vi "ShooterManualFlyWheel.vi"(11 "Cluster":T1) -> ()   [LabVIEW 2015]
doc: "call on constants for shooting and give them to the respective motors"
uses:
  constants/constants.ctl
  <vilib>/Rock Robotics/SystemInterfaces/DIO/FPGA_DIOPWMChannel.ctl
  <vilib>/Rock Robotics/WPI/Solenoid/WPI_SolenoidChannel.ctl
panel:
  # "ShooterMotors"
  # "DriveMotors- CAN Bus"
  # "PWM"
  # "ClimberMotors"
  # "CAN Bus"
  # "Pnematic"
  # "PWM"
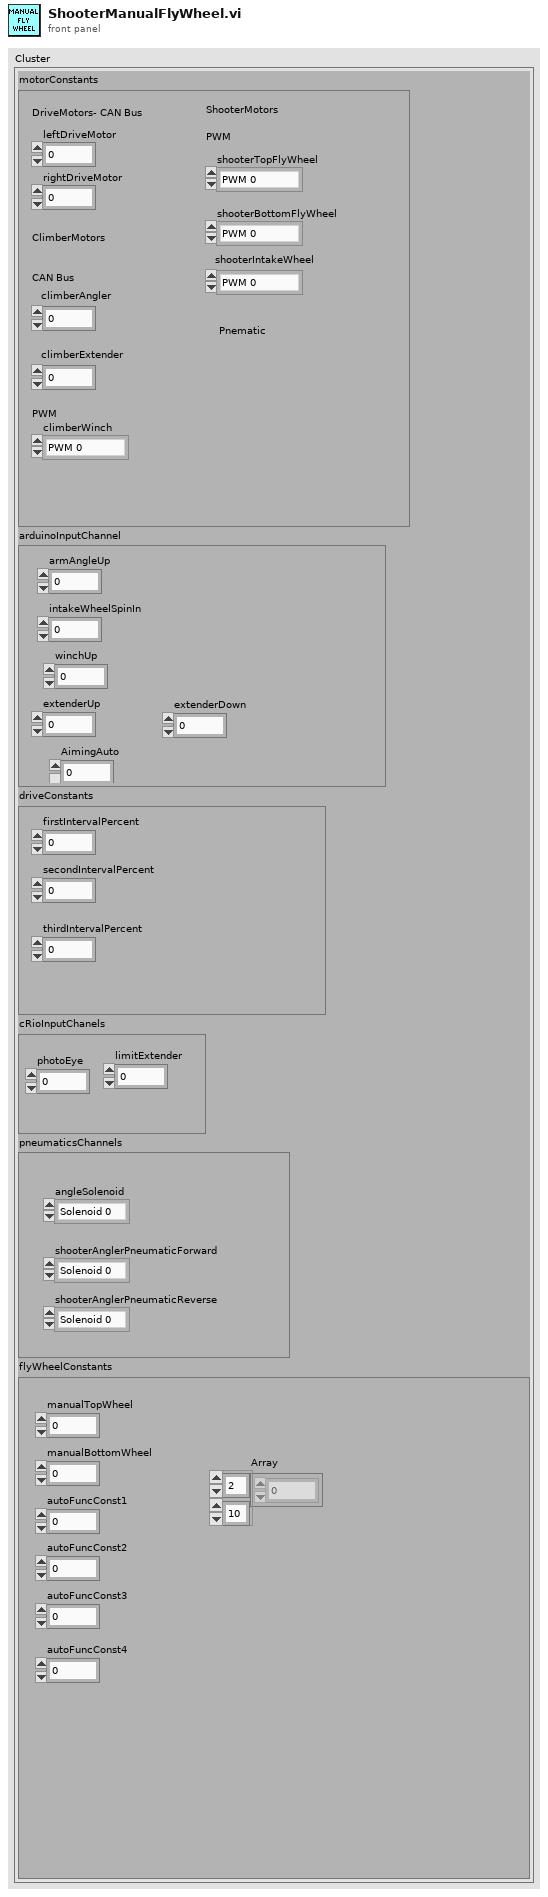
[diagram p1: front panel]
types:
  T1 = typedef "constants.ctl" = cluster{"motorConstants":cluster{"leftDriveMotor":i32, "rightDriveMotor":i32, "climberAngler":i32, "climberWinch":T2, "shooterTopFlyWheel":T2, "shooterBottomFlyWheel":T2, "climberExtender":i32, "shooterIntakeWheel":T2}, "arduinoInputChannel":cluster{"armAngleUp":i32, "intakeWheelSpinIn":i32, "winchUp":i32, "extenderUp":i32, "AimingAuto":i32, "extenderDown":i32}, "driveConstants":cluster{"firstIntervalPercent":dbl, "secondIntervalPercent":dbl, "thirdIntervalPercent":dbl}, "cRioInputChanels":cluster{"photoEye":i32, "limitExtender":i32}, "pneumaticsChannels":cluster{"angleSolenoid":T3, "shooterAnglerPneumaticForward":T3, "shooterAnglerPneumaticReverse":T3}, "flyWheelConstants":cluster{"manualTopWheel":dbl, "manualBottomWheel":dbl, "autoFuncConst1":dbl, "autoFuncConst2":dbl, "autoFuncConst3":dbl, "autoFuncConst4":dbl, "Array":dbl[][]}}
  T2 = typedef "FPGA_DIOPWMChannel.ctl" = enum8{"PWM 0", "PWM 1", "PWM 2", "PWM 3", "PWM 4", "PWM 5", "PWM 6", "PWM 7", "PWM 8", "PWM 9", "PWM MXP 0", "PWM MXP 1", "PWM MXP 2", "PWM MXP 3", "PWM MXP 4", "PWM MXP 5", "PWM MXP 6", "PWM MXP 7", "PWM MXP 8", "PWM MXP 9", "Invalid"}
  T3 = typedef "WPI_SolenoidChannel.ctl" = enum8{"Solenoid 0", "Solenoid 1", "Solenoid 2", "Solenoid 3", "Solenoid 4", "Solenoid 5", "Solenoid 6", "Solenoid 7", "Invalid"}
  T4 = typedef "WPI_MotorControlDeviceRef.ctl" = cluster{"DeviceStatus":errorcluster, "Type":T5, "PWM":cluster{"PWM Channel":T2, "DeadBand":T6}, "CAN":cluster{"Device Number":u8, "Control Mode":T7, "Semaphore":T8, "Max Vout":dbl, "TalonSRX Control Mode":T9}, "Invert":bool}
  T5 = typedef "WPI_MotorControlType.ctl" = enum16{"PWM", "CAN", "CANTalonSRX"}
  T6 = typedef "WPI_PWMDeadband.ctl" = cluster{"Name":string, "maxPositivePwm":i32, "minPositivePwm":i32, "centerPwm":i32, "maxNegativePwm":i32, "minNegativePwm":i32, "angularRange":u16}
  T7 = typedef "WPI_CANJaguar_ControlMode.ctl" = enum8{"Percent VBus", "Current", "Speed", "Position", "Voltage"}
  T8 = typedef "Semaphore RefNum" = refnum<k1>
  T9 = typedef "WPI_CANTalonSRX_APIControlMode.ctl" = enum8{"Percent VBus", "Speed", "Position", "Slave", "Unchanged / Invalid", "Voltage Compensation", "Current", "Motion Profile"}
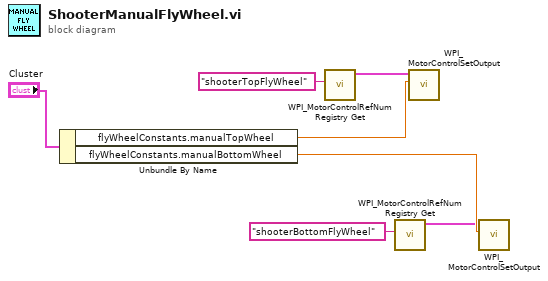
[diagram p0: block diagram]
diagram:
  n1 = Unbundle By Name("Cluster") -> ("flyWheelConstants.manualTopWheel"=w6:dbl, "flyWheelConstants.manualBottomWheel"=w7:dbl)
  n2 = call <vilib>:"WPI_MotorControlRefNum Registry Get.vi"("refnum name"="shooterTopFlyWheel") -> ("MotorControlDevRef"=w2:T4)  [unwired: 9 in, 1 out]
  n3 = call <vilib>:"WPI_MotorControlRefNum Registry Get.vi"("refnum name"="shooterBottomFlyWheel") -> ("MotorControlDevRef"=w4:T4)  [unwired: 9 in, 1 out]
  n4 = call <vilib>:"WPI_MotorControlSetOutput.vi"("Output"=w6, "MotorControlDevRef"=w2) -> ()  [unwired: 7 in, 3 out]
  n5 = call <vilib>:"WPI_MotorControlSetOutput.vi"("Output"=w7, "MotorControlDevRef"=w4) -> ()  [unwired: 7 in, 3 out]
